vi "Send Callback Message.vi"(8 "error in (no error)":errorcluster, 11 "Order Item in":refnum<class "Order Item.lvclass">) -> (0 "error out":errorcluster, 3 "Order Item out":refnum<class "Order Item.lvclass">)   [LabVIEW 2020, in "Order Item.lvclass"]
doc: "Send the callback message provided by the caller. This enables a zero-coupling relationship between the caller and the callee."
uses:
  Order Item.lvclass
  Pick Up Order/Pick Up Order.lvclass
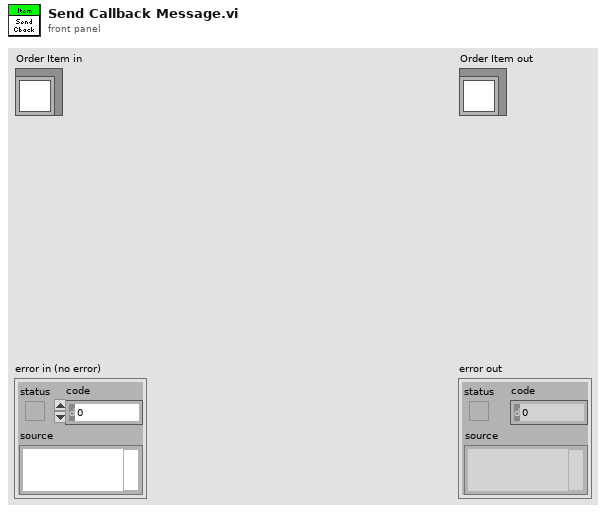
[diagram p1: front panel]
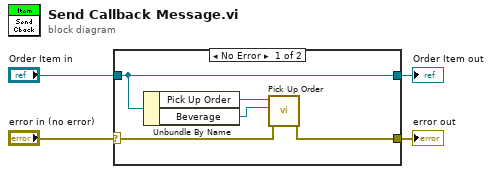
[diagram p0: block diagram]
diagram:
  n1 = case shown="No Error" "error in (no error)" {
    selector: "error in (no error)" -> [w7 w11]
    tunnel: [w6 w11] -> w3
    tunnel: [w9 w10] -> w1
    tunnel: "Order Item in" -> [w9 w10]
    frame No Error {
      n2 = Unbundle By Name(w9) -> ("Pick Up Order"=w8:refnum<class "Pick Up Order.lvclass">, "Beverage"=w5:refnum<class "Beverage.lvclass">)
      n3 = call-dynamic "Pick Up Order.vi"("error in (no error)"=w7, "Beverage"=w5, "Pick Up Order in"=w8) -> ("error out"=w6:errorcluster)  [unwired: 7 in, 1 out]
    }
    frame Error {
    }
  }
  "error out" <- w3
  "Order Item out" <- w1
